vi "read TBM configuration.vi"(8 "error in":errorcluster, 11 "tag bus configurable plugin editor node in":refnum<class "TEST EDITOR.lvclass">) -> (0 "error out":errorcluster, 2 "configuration":refnum<class "TBM configuration.lvclass">, 3 "tag bus configurable plugin editor node out":refnum<class "TEST EDITOR.lvclass">)   [LabVIEW 2013, in "configuration tests.lvlib" / "TEST EDITOR.lvclass"]
uses:
  TEST EDITOR.lvclass
  <vilib>/NI/Tag Bus Module Framework/root configuration/TBM configuration.lvclass
  TEST EDITOR.lvclass/TEST EDITOR.ctl
  module/configuration/TEST CONFIGURATION.lvclass
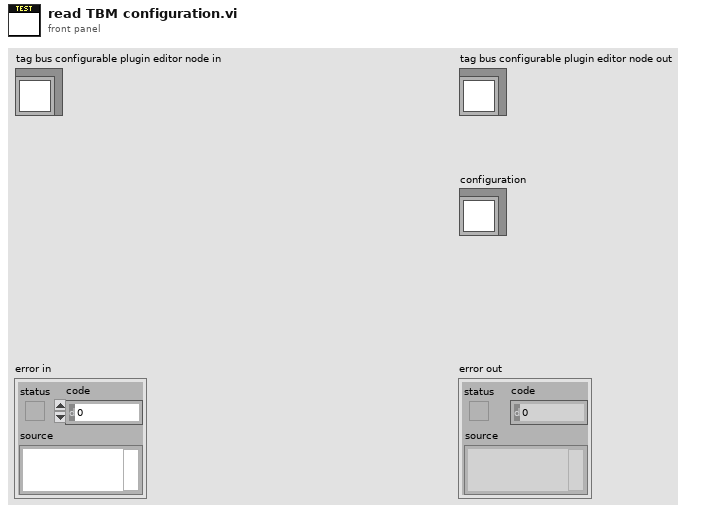
[diagram p1: front panel]
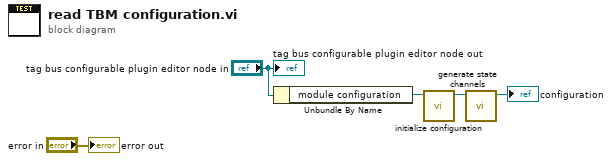
[diagram p0: block diagram]
diagram:
  n1 = Unbundle By Name("tag bus configurable plugin editor node in") -> ("module configuration"=w3:refnum<class "TEST CONFIGURATION.lvclass">)
  n2 = call-dynamic "initialize configuration.vi"("configuration in"=w3) -> ("configuration out"=w1:refnum<class "TEST CONFIGURATION.lvclass">)  [unwired: 8 in, 2 out]
  n3 = call "generate state channels.vi"("tag bus configurable plugin module configuration in"=w1) -> ("tag bus configurable plugin module configuration out"=→"configuration":refnum<class "TEST CONFIGURATION.lvclass">)  [unwired: 9 in, 1 out]
  "error out" <- "error in"
  "tag bus configurable plugin editor node out" <- "tag bus configurable plugin editor node in"
